vi "Thev-Compute Zx.vi"(0 "Zs":cdb[](array[numeric]), 5 "Ps":cdb[](array[numeric]), 7 "Px":cdb[](array[numeric])) -> (8 "Zx":cdb[](array[numeric]))   [LabVIEW 2015]
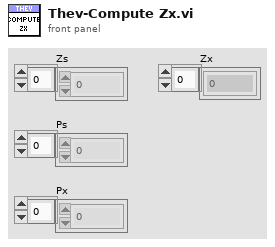
[diagram p1: front panel]
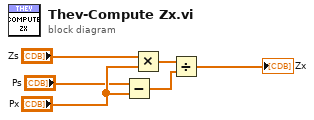
[diagram p0: block diagram]
diagram:
  n1 = Subtract(x="Ps", y="Px") -> (x-y=w1:cdb[])
  n2 = Multiply(x="Zs", y="Px") -> (x*y=w2:cdb[])
  n3 = Divide(x=w2, y=w1) -> (x/y=→"Zx":cdb[])
